vi "Write action name.vi"(8 "error in (no error)":errorcluster, 10 "action name":string, 11 "RenameVIsandClasses in":refnum<class "SequencerActionScript.lvclass">) -> (0 "error out":errorcluster, 3 "RenameVIsandClasses out":refnum<class "SequencerActionScript.lvclass">)   [LabVIEW 2014, in "SequencerActionScript.lvclass"]
uses:
  SequencerActionScript.lvclass
  SequencerActionScript.lvclass/SequencerActionScript.ctl
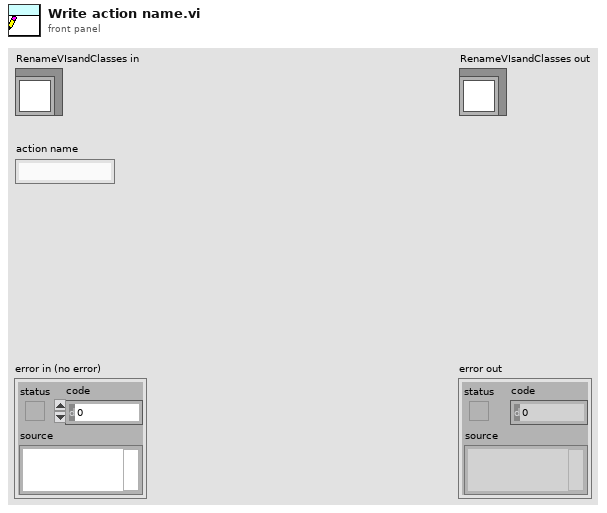
[diagram p1: front panel]
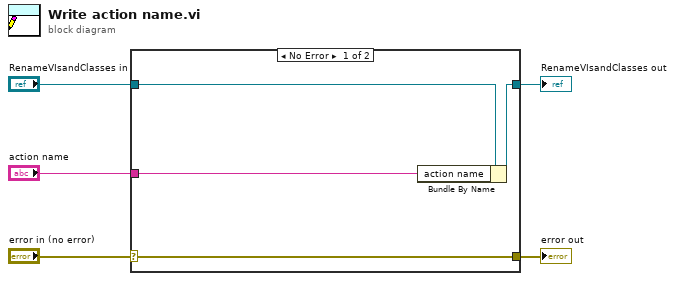
[diagram p0: block diagram]
diagram:
  n1 = case shown="No Error" "error in (no error)" {
    selector: "error in (no error)" -> [w9 w10]
    tunnel: [w9 w10] -> w4
    tunnel: [w7 w11] -> w2
    tunnel: "RenameVIsandClasses in" -> [w8 w11]
    tunnel: "action name" -> [w6 _]
    frame No Error {
      n2 = Bundle By Name(cluster=w8, "action name"=w6) -> (w7:refnum<class "SequencerActionScript.lvclass">)
    }
    frame Error {
    }
  }
  "error out" <- w4
  "RenameVIsandClasses out" <- w2
